vi "Day06-1.vi"() -> ()   [LabVIEW 2021]
panel:
  out "fish":i32
  out "Day":i32
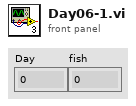
[diagram p1: front panel]
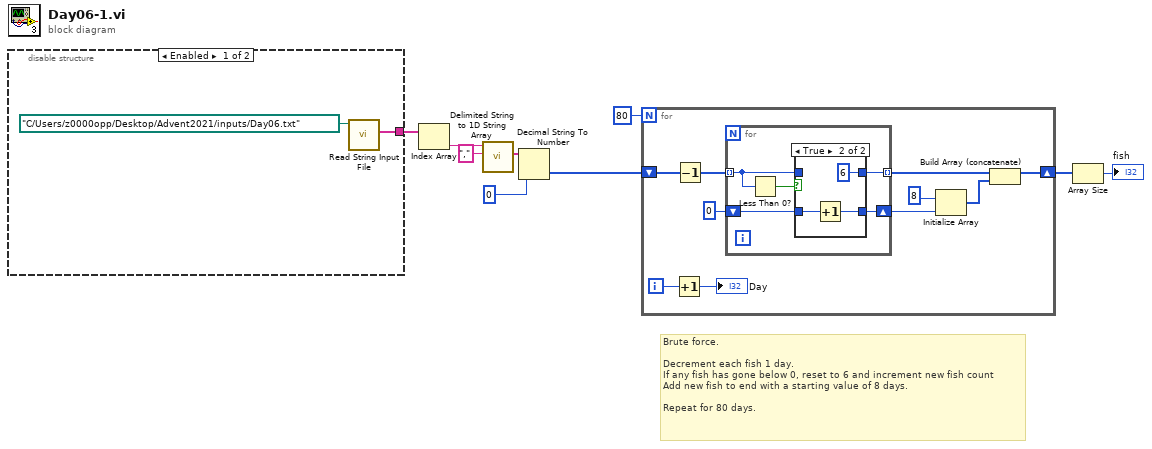
[diagram p0: block diagram]
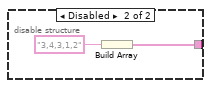
[diagram p3: hidden frame]
diagram:
  # "Brute force.\n\nDecrement each fish 1 day.\nIf any fish has gone below 0, reset to 6 and increment new fish count\nAdd new fish to end with a starting value of 8 days.\n\nRepeat for 80 days."
  n1 = disable-structure shown="Enabled" {
    disable-tunnel: [w10 w12] -> w8
    frame Enabled {
      n2 = call "Read String Input File.vi"("file path (dialog if empty)"=path "C:/Users/z0000opp/Desktop/Advent2021/inputs/Day06.txt") -> ("input values"=w10:string[])  [unwired: 10 in]
    }
    frame Disabled {
      n3 = Build Array("3,4,3,1,2") -> (w12:string[])
    }
  }
  n4 = Index Array(array=w8) -> (element=w7:string)  [unwired: 1 in]
  n5 = call <vilib>:"Delimited String to 1D String Array.vi"("delimiter"=",", "delimited string"=w7) -> ("string array"=w9:string[])  [unwired: 9 in]
  n6 = Decimal String To Number(string=w9, default (0L)=i64 0) -> (number=w5:i64[])  [unwired: 1 in, 1 out]
  n7 = for {
    N: 80 -> [_]
    shift-right: [w14] -> w3
    shift-left: w5 -> [w23]
    i -> [w20]
    n8 = Increment(x=w20) -> (x+1=→"Day":i32)
    n9 = Decrement(x=w23) -> (x-1=w22:i64[])
    n10 = for {
      tunnel: w22 -> [w27] mode=indexing
      shift-right: [w24] -> w18
      shift-left: 0 -> [w25]
      tunnel: [w26] -> w16 mode=indexing
      n11 = Less Than 0?(x=w27) -> (x < 0?=w28:bool)
      n12 = case shown="True" w28 {
        tunnel: w27 -> [w30 _]
        tunnel: [w30 i64 6 ("String")] -> w26
        tunnel: w25 -> [w29 w32]
        tunnel: [w29 w31] -> w24
        frame False {
        }
        frame True {
          n13 = Increment(x=w32) -> (x+1=w31:i32)
        }
      }
    }
    n14 = Initialize Array(i64 8, w18) -> (w15:i64[])
    n15 = Build Array (concatenate)(w16, w15) -> (w14:i64[])
  }
  n16 = Array Size(array=w3) -> (size(s)=→"fish":i32)
